vi "CAN_getOutput.vi"(8 "error in (no error)":errorcluster, 11 "CAN Jaguars Ref":T1) -> (0 "error out":errorcluster, 1 "Right output":dbl, 2 "Left output":dbl, 3 "CAN Jaguars Ref out":T1)   [LabVIEW 2009, in "OWNCAN.lvlib"]
uses:
  OWNCAN.lvlib
  CAN Jaguars Ref.ctl
  CAN/SubVIs/CAN Jaguar Ref.ctl
  CAN/SubVIs/CAN Jaguar Control Mode.ctl
  CAN/SubVIs/CAN Jaguar Status Select.ctl
  CAN.lvlib
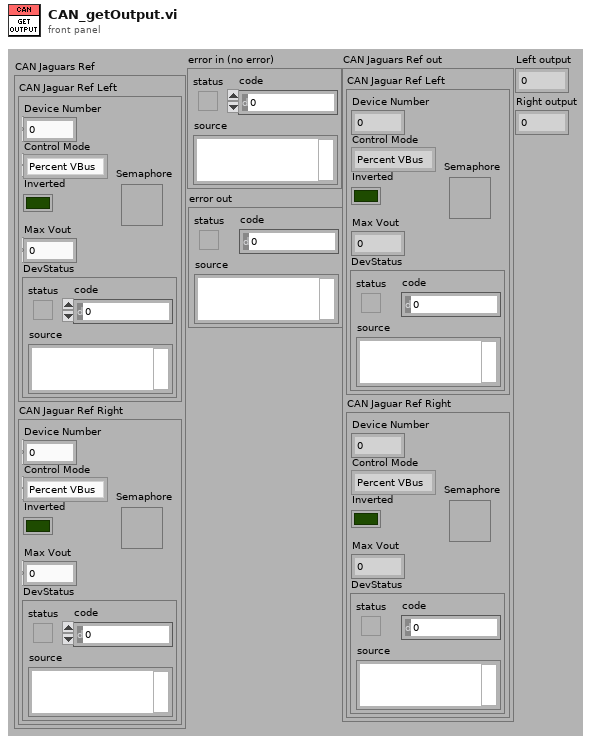
[diagram p1: front panel]
types:
  T1 = typedef "OWNCAN.lvlib/CAN Jaguars Ref.ctl" = cluster{"CAN Jaguar Ref Left":T2, "CAN Jaguar Ref Right":T2}
  T2 = typedef "CAN.lvlib/CAN Jaguar Ref.ctl" = cluster{"Device Number":u8, "Control Mode":T3, "Inverted":bool, "Semaphore":T4, "Max Vout":dbl, "DevStatus":errorcluster}
  T3 = typedef "CAN.lvlib/CAN Jaguar Control Mode.ctl" = enum16{"Percent VBus", "Speed", "Position", "Current"}
  T4 = typedef "Semaphore RefNum" = refnum<k1>
  T5 = typedef "CAN.lvlib/CAN Jaguar Status Select.ctl" = enum16{"Voltage", "Current", "Temperature", "Position", "Speed", "Limit Switches", "Faults", "Power Cycle"}
  T6 = typedef "CAN.lvlib/CAN Jaguar Status.ctl" = cluster{"Output Voltage":dbl, "Bus Voltage":dbl, "Current":dbl, "Temperature":dbl, "Position":dbl, "Speed":dbl, "Forward Limit":bool, "Reverse Limit":bool, "Current Fault":bool, "Temperature Fault":bool, "Bus Voltage Fault":bool, "Power Cycle":bool}
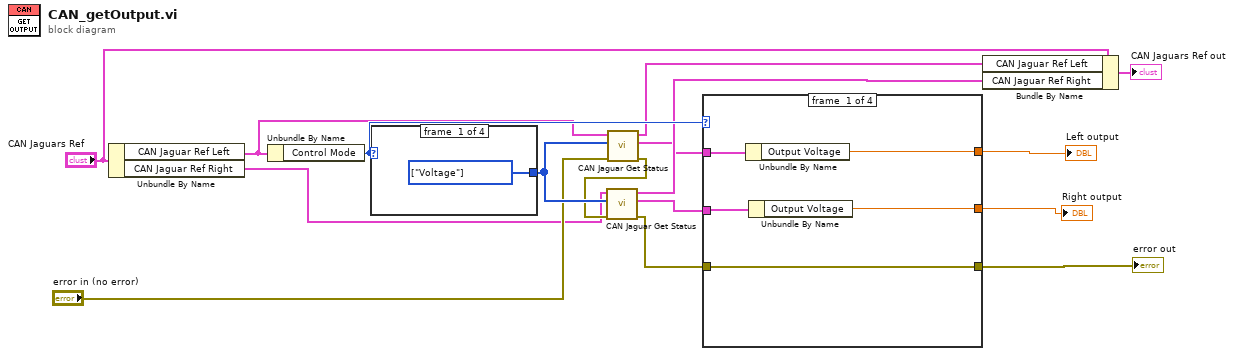
[diagram p0: block diagram]
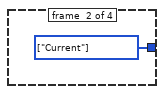
[diagram p2: hidden frame]
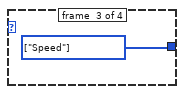
[diagram p3: hidden frame]
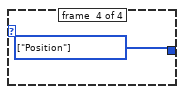
[diagram p4: hidden frame]
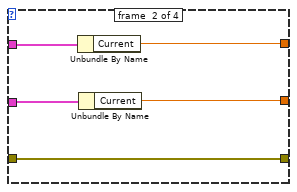
[diagram p5: hidden frame]
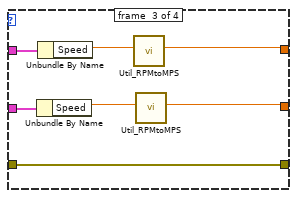
[diagram p6: hidden frame]
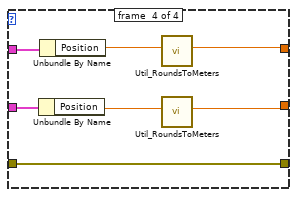
[diagram p7: hidden frame]
diagram:
  n1 = Unbundle By Name("CAN Jaguars Ref") -> ("CAN Jaguar Ref Left"=w11:T2, "CAN Jaguar Ref Right"=w10:T2)
  n2 = Unbundle By Name(w11) -> ("Control Mode"=w12:T3)
  n3 = case shown="\"Current\"" w12 {
    tunnel: [w17 w18 w19 w20] -> w16
    frame #0 {
      w17 = T5[] [enum."Voltage"] items=["Voltage", "Current", "Temperature", "Position", "Speed", "Limit Switches", "Faults", "Power Cycle"] ("Status Select")
    }
    frame #1 {
      w18 = T5[] [enum."Current"] items=["Voltage", "Current", "Temperature", "Position", "Speed", "Limit Switches", "Faults", "Power Cycle"] ("Status Select")
    }
    frame #2 {
      w19 = T5[] [enum."Speed"] items=["Voltage", "Current", "Temperature", "Position", "Speed", "Limit Switches", "Faults", "Power Cycle"] ("Status Select")
    }
    frame #3 {
      w20 = T5[] [enum."Position"] items=["Voltage", "Current", "Temperature", "Position", "Speed", "Limit Switches", "Faults", "Power Cycle"] ("Status Select")
    }
  }
  n4 = call "CAN Jaguar Get Status.vi"("error in (no error)"="error in (no error)", "Status Select"=w16, "CAN Jaguar Ref"=w11) -> ("error out"=w14:errorcluster, "Status"=w6:T6, "CAN Jaguar Ref Out"=w8:T2)  [unwired: 6 in]
  n5 = call "CAN Jaguar Get Status.vi"("error in (no error)"=w14, "Status Select"=w16, "CAN Jaguar Ref"=w10) -> ("error out"=w13:errorcluster, "Status"=w5:T6, "CAN Jaguar Ref Out"=w7:T2)  [unwired: 6 in]
  n6 = case shown="\"Speed\"" w12 {
    tunnel: w13 -> [w21 w26 w31 w38]
    tunnel: w6 -> [w25 w30 w37 w44]
    tunnel: w5 -> [w24 w29 w36 w43]
    tunnel: [w23 w28 w34 w41] -> w2
    tunnel: [w22 w27 w32 w39] -> w1
    tunnel: [w21 w26 w31 w38] -> w3
    frame #0 {
      n7 = Unbundle By Name(w25) -> ("Output Voltage"=w23:dbl)
      n8 = Unbundle By Name(w24) -> ("Output Voltage"=w22:dbl)
    }
    frame #1 {
      n9 = Unbundle By Name(w30) -> ("Current"=w28:dbl)
      n10 = Unbundle By Name(w29) -> ("Current"=w27:dbl)
    }
    frame #2 {
      n11 = Unbundle By Name(w36) -> ("Speed"=w33:dbl)
      n12 = Unbundle By Name(w37) -> ("Speed"=w35:dbl)
      n13 = call "Util_RPMtoMPS.vi"("rpm gear"=w35) -> ("m/s robot"=w34:dbl)  [unwired: 10 in]
      n14 = call "Util_RPMtoMPS.vi"("rpm gear"=w33) -> ("m/s robot"=w32:dbl)  [unwired: 10 in]
    }
    frame #3 {
      n15 = Unbundle By Name(w43) -> ("Position"=w40:dbl)
      n16 = Unbundle By Name(w44) -> ("Position"=w42:dbl)
      n17 = call "Util_RoundsToMeters.vi"("rounds gear"=w42) -> ("distance (m) robot"=w41:dbl)  [unwired: 10 in]
      n18 = call "Util_RoundsToMeters.vi"("rounds gear"=w40) -> ("distance (m) robot"=w39:dbl)  [unwired: 10 in]
    }
  }
  "error out" <- w3
  "Left output" <- w2
  "Right output" <- w1
  n19 = Bundle By Name(cluster="CAN Jaguars Ref", "CAN Jaguar Ref Left"=w8, "CAN Jaguar Ref Right"=w7) -> (→"CAN Jaguars Ref out":T1)
